vi "Spin pumping 83650B-2182-Kepco-475.vi"() -> ()   [LabVIEW 2020]
uses:
  <vilib>/Utility/file.llb/Write Delimited Spreadsheet (DBL).vi
panel:
  out "appended path":path
  in  "File Name":string
  in  "error out":errorcluster
  in  "stop":bool
  in  "Model 475 GPIB Addr":string="14"
  in  "Kepco GPIB Addr":string="6"
  in  "Model 2182 GPIB Addr":string="7"
  in  "83650B GPIB Addr":string="19"
  in  "Measurement Selection":T1(tab)
  out "History":cluster{dbl[], dbl[]}(graph)
  in  "Task":string[][](table)=[["1", "15", "8", "0.05", "2"]]
  out "Ongoing Measurement":cluster{dbl[], dbl[]}(graph)
  in  "Run":bool
  out "History 2":cluster{dbl[], dbl[]}(graph)
  in  "Task 2":string[][](table)=[["4", "1", "5", "0.05", "15", "10"]]
  out "Ongoing Measurement 2":cluster{dbl[], dbl[]}(graph)
  in  "Run 2":bool
  out "Field (Oe)":dbl
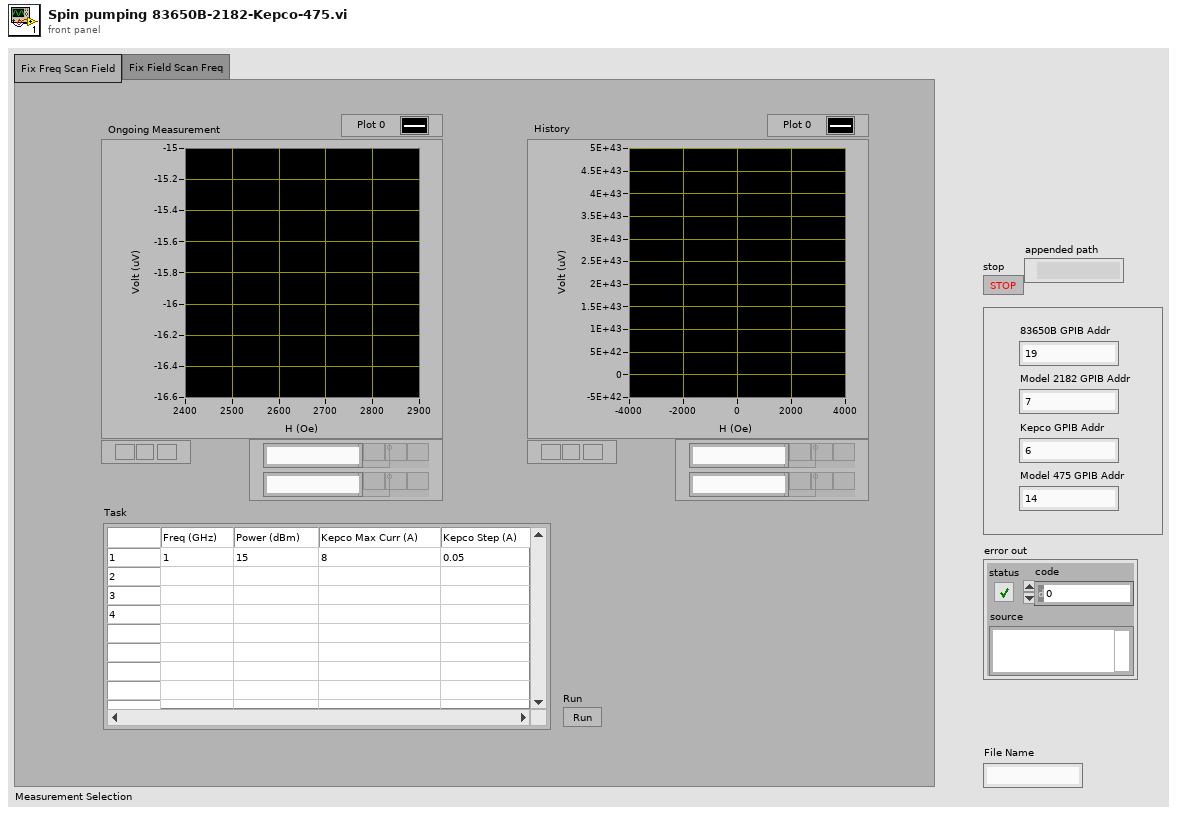
[diagram p1: front panel]
types:
  T1 = enum32{"Fix Freq Scan Field", "Fix Field Scan Freq"}
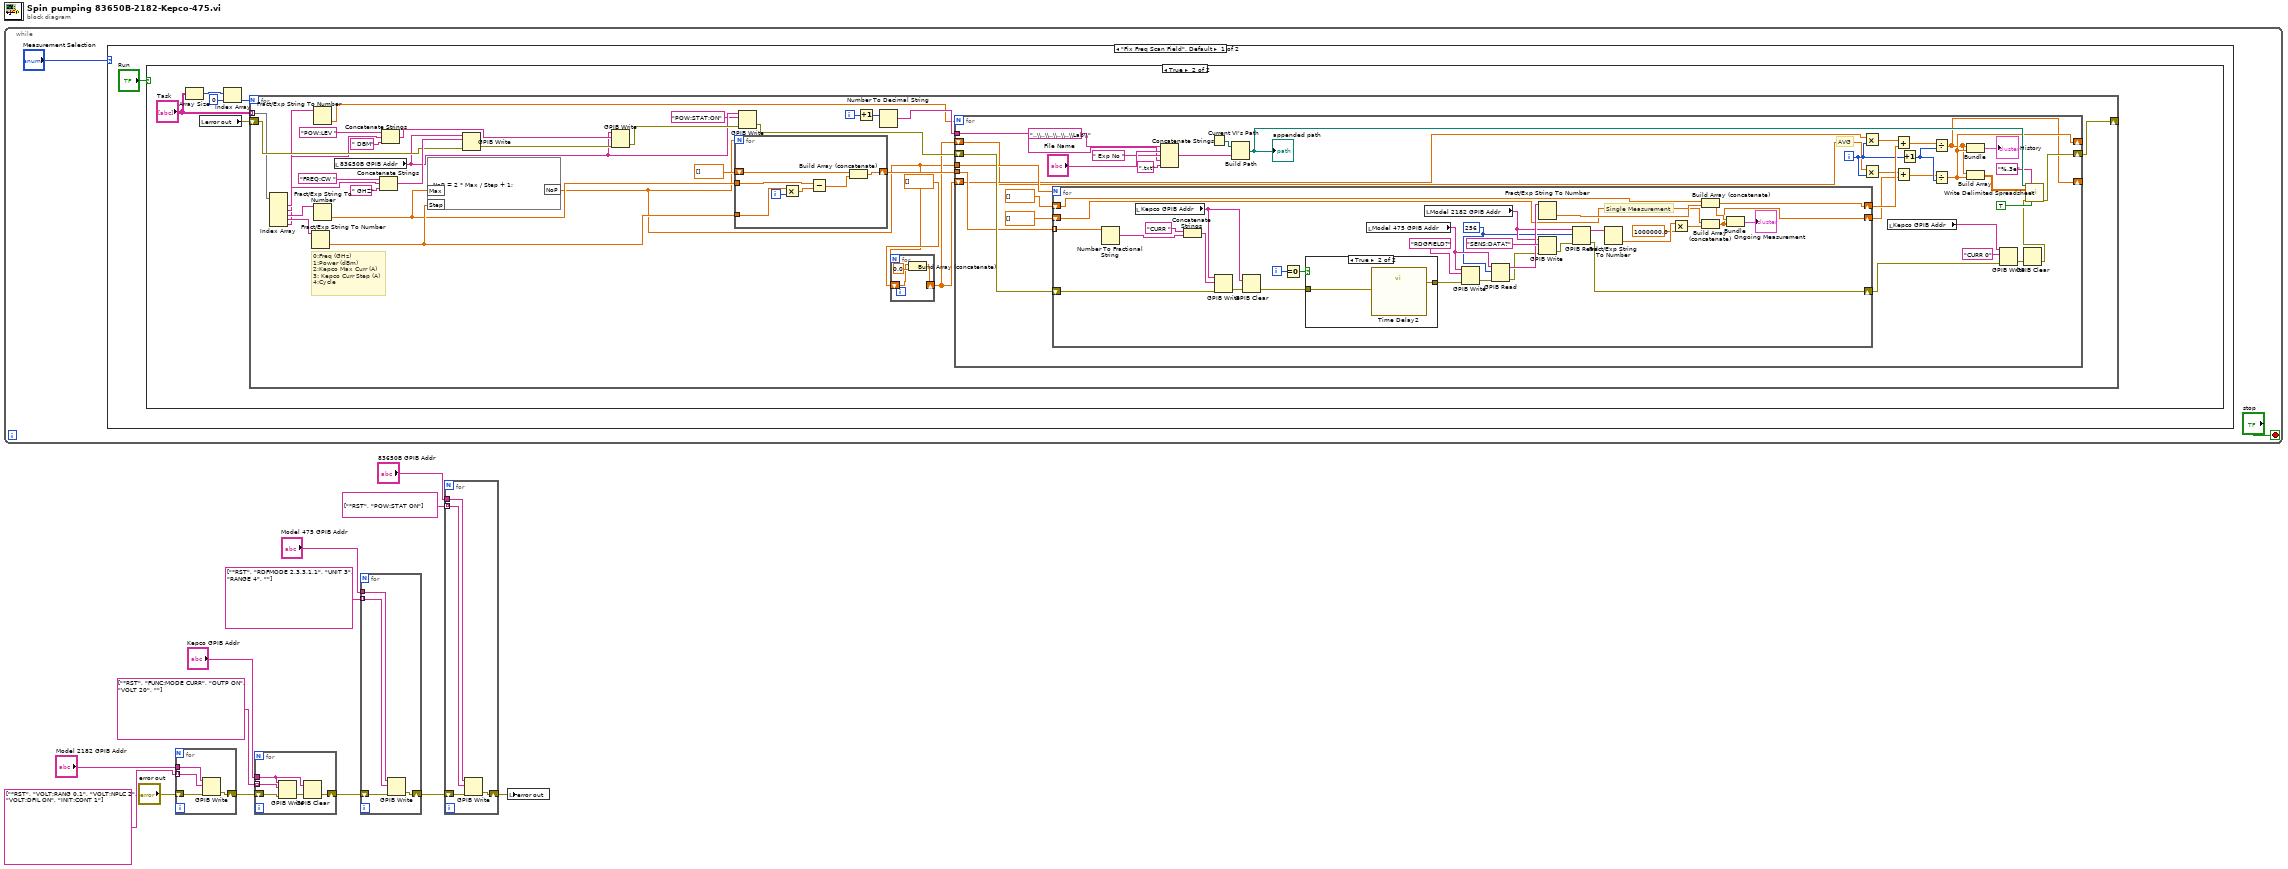
[diagram p0: block diagram]
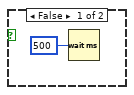
[diagram p2: hidden frame]
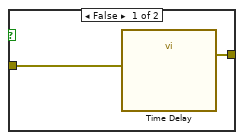
[diagram p3: hidden frame]
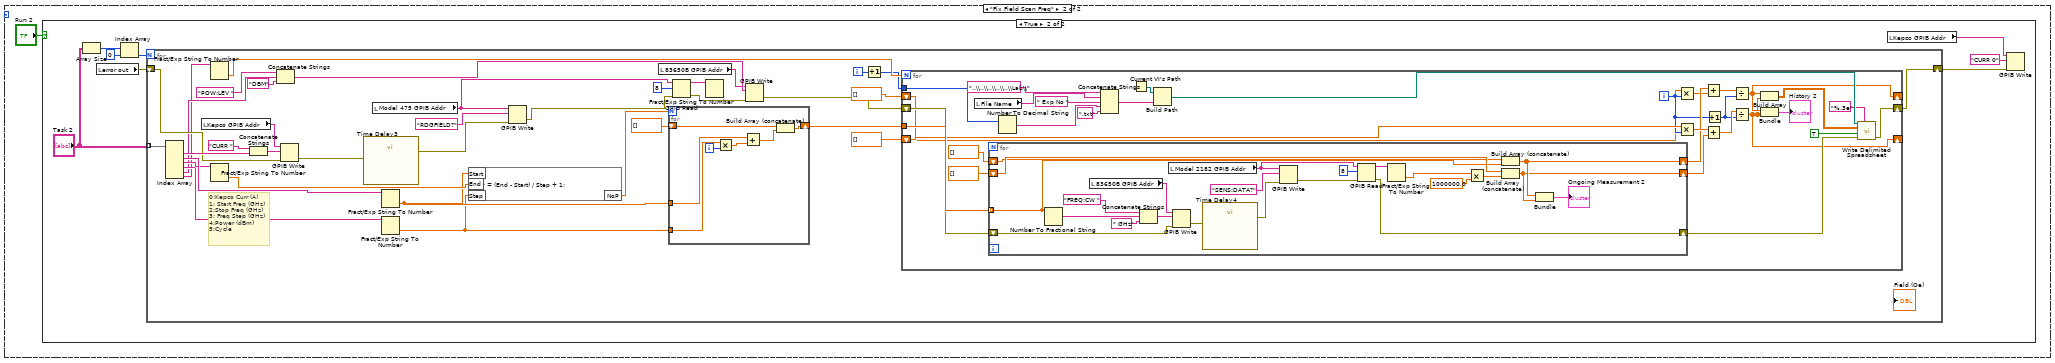
[diagram p4: hidden frame]
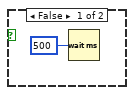
[diagram p5: hidden frame]
diagram:
  n1 = while {
    stop <- "stop" stop-if-true
    n2 = case shown="\"Fix Freq Scan Field\", Default" "Measurement Selection" {
      frame "Fix Freq Scan Field", Default {
        n3 = case shown="True" "Run" {
          frame False {
            n4 = Wait (ms)(milliseconds to wait=u32 500) -> ()  [unwired: 1 out]
          }
          frame True {
            n5 = Array Size(array="Task") -> (size(s)=w22:i32[])
            n6 = local read "error out"() -> (w18:errorcluster)
            n7 = Index Array(array=w22, index=0) -> (element=w21:i32)
            n8 = for {
              N: w21 -> [_]
              tunnel: "Task" -> [w40] mode=indexing
              shift-right: [w34] -> _
              shift-left: w18 -> [w42]
              i -> [w33]
              # "0:Freq (GHz)\n1:Power (dBm)\n2:Kepco Max Curr (A)\n3: Kepco Curr Step (A)\n4:Cycle"
              n9 = Index Array(array=w40) -> (element #1=w41:string, element #2=w39:string, element #3=w38:string, element #4=w37:string, element #5=w36:string)  [unwired: 5 in]
              n10 = Fract/Exp String To Number(string=w37) -> (number=w45:dbl)  [unwired: 3 in, 1 out]
              n11 = Fract/Exp String To Number(string=w36) -> (number=w26:dbl)  [unwired: 3 in, 1 out]
              n12 = Fract/Exp String To Number(string=w38) -> (number=w44:dbl)  [unwired: 3 in, 1 out]
              n13 = local read "83650B GPIB Addr"() -> (w28:string)
              n14 = Concatenate Strings("FREQ:CW " ("string"), w41, " GHZ" ("string")) -> (w48:string)
              n15 = Concatenate Strings("POW:LEV " ("string"), w39, " DBM" ("string")) -> (w50:string)
              n16 = formula code="NoP = 2 * Max / Step + 1;"("Max"=w44, "Step"=w45) -> ("NoP"=w23:dbl)
              n17 = GPIB Write(0:w28, 1:w48, 3:w42) -> (6:w49:errorcluster)  [unwired: 2 in, 1 out]
              n18 = GPIB Write(0:w28, 1:w50, 3:w49) -> (6:w29:errorcluster)  [unwired: 2 in, 1 out]
              n19 = for {
                N: w23 -> [_]
                shift-right: [w126] -> w35
                shift-left: dbl[] [] -> [w127]
                tunnel: w45 -> [w131]
                tunnel: w44 -> [w129]
                i -> [w132]
                n20 = Multiply(x=w131, y=w132) -> (x*y=w130:dbl)
                n21 = Subtract(x=w129, y=w130) -> (x-y=w128:dbl)
                n22 = Build Array (concatenate)(w127, w128) -> (w126:dbl[])
              }
              n23 = GPIB Write(0:w28, 1:"POW:STAT:ON" ("data"), 3:w29) -> (6:w30:errorcluster)  [unwired: 2 in, 1 out]
              n24 = Increment(x=w33) -> (x+1=w32:i32)
              n25 = Number To Decimal String(number=w32) -> (decimal integer string=w31:string)  [unwired: 1 in]
              n26 = for {
                N: w23 -> [_]
                shift-right: [w53] -> w24
                shift-left: dbl[] [] -> [w54]
                n27 = Build Array (concatenate)(w54, 0.0 ("element")) -> (w53:dbl[])
              }
              n28 = for {
                N: w26 -> [_]
                shift-right: [w81] -> w34
                shift-left: w30 -> [w84]
                tunnel: w35 -> [w83]
                tunnel: w23 -> [w82]
                shift-right: [w68] -> _
                shift-left: w24 -> [w77]
                shift-right: [w69] -> _
                shift-left: w24 -> [w72]
                tunnel: w31 -> [w63]
                i -> [w73]
                # "AVG"
                n29 = for {
                  N: w82 -> [_]
                  shift-right: [w102] -> w57
                  shift-left: w84 -> [w121]
                  tunnel: w83 -> [w119] mode=indexing
                  shift-right: [w101] -> w80
                  shift-left: dbl[] [] -> [w108]
                  shift-right: [w100] -> w75
                  shift-left: dbl[] [] -> [w104]
                  i -> [w114]
                  w106 = 256 ("byte count")
                  # "Single Measurement"
                  n30 = Number To Fractional String(number=w119) -> (F-format string=w118:string)  [unwired: 3 in]
                  n31 = local read "Kepco GPIB Addr"() -> (w91:string)
                  n32 = Concatenate Strings("CURR " ("string"), w118) -> (w117:string)
                  n33 = GPIB Write(0:w91, 1:w117, 3:w121) -> (6:w93:errorcluster)  [unwired: 2 in, 1 out]
                  n34 = GPIB Clear(2:w93, 3:w91) -> (0:w92:errorcluster)  [unwired: 1 out]
                  n35 = Equal To 0?(x=w114) -> (x = 0?=w113:bool)
                  n36 = case shown="True" w113 {
                    tunnel: w92 -> [w123 w125]
                    tunnel: [w122 w124] -> w115
                    frame False {
                      n37 = call "Time Delay"("error in (no error)"=w123) -> ("error out"=w122:errorcluster)  [unwired: 10 in]
                    }
                    frame True {
                      n38 = call "Time Delay2"("error in (no error)"=w125) -> ("error out"=w124:errorcluster)  [unwired: 10 in]
                    }
                  }
                  n39 = local read "Model 475 GPIB Addr"() -> (w111:string)
                  n40 = local read "Model 2182 GPIB Addr"() -> (w107:string)
                  n41 = GPIB Write(0:w111, 1:"RDGFIELD?" ("data"), 3:w115) -> (6:w95:errorcluster)  [unwired: 2 in, 1 out]
                  n42 = GPIB Read(0:w111, 1:w106, 3:w95) -> (5:w110:string, 7:w94:errorcluster)  [unwired: 2 in, 1 out]
                  n43 = Fract/Exp String To Number(string=w110) -> (number=w109:dbl)  [unwired: 3 in, 1 out]
                  n44 = GPIB Write(0:w107, 1:"SENS:DATA?" ("data"), 3:w94) -> (6:w103:errorcluster)  [unwired: 2 in, 1 out]
                  n45 = GPIB Read(0:w107, 1:w106, 3:w103) -> (5:w105:string, 7:w102:errorcluster)  [unwired: 2 in, 1 out]
                  n46 = Fract/Exp String To Number(string=w105) -> (number=w98:dbl)  [unwired: 3 in, 1 out]
                  n47 = Multiply(x=w98, y=1000000.0) -> (x*y=w96:dbl)
                  n48 = Build Array (concatenate)(w108, w109) -> (w101:dbl[])
                  n49 = Build Array (concatenate)(w104, w96) -> (w100:dbl[])
                  n50 = Bundle(w101, w100) -> (→"Ongoing Measurement":cluster{dbl[], dbl[]})  [unwired: 1 in]
                }
                n51 = Concatenate Strings("..\\..\\..\\..\\..\\Lab\\" ("string"), "File Name", " Exp No " ("string"), w63, ".txt" ("string")) -> (w88:string)
                n52 = Current VI's Path() -> (path=w62:path)
                n53 = Build Path(base path=w62, name or relative path=w88) -> (appended path=w89:path)
                "appended path" <- w89
                n54 = Multiply(x=w77, y=w73) -> (x*y=w79:dbl[])
                n55 = Multiply(x=w72, y=w73) -> (x*y=w74:dbl[])
                n56 = local read "Kepco GPIB Addr"() -> (w59:string)
                n57 = Add(x=w79, y=w80) -> (x+y=w78:dbl[])
                n58 = Add(x=w74, y=w75) -> (x+y=w71:dbl[])
                n59 = Increment(x=w73) -> (x+1=w76:i32)
                n60 = Divide(x=w78, y=w76) -> (x/y=w68:dbl[])
                n61 = Divide(x=w71, y=w76) -> (x/y=w69:dbl[])
                n62 = Bundle(w68, w69) -> (→"History":cluster{dbl[], dbl[]})  [unwired: 1 in]
                n63 = Build Array(w68, w69) -> (w67:dbl[][])
                n64 = GPIB Write(0:w59, 1:"CURR 0" ("data"), 3:w57) -> (6:w60:errorcluster)  [unwired: 2 in, 1 out]
                n65 = GPIB Clear(2:w60) -> (0:w56:errorcluster)  [unwired: 1 in, 1 out]
                n66 = call-poly <vilib>:"Write Delimited Spreadsheet.vi"("file path (dialog if empty)"=w89, "format (%.3f)"="%.3e", "2D data"=w67, "error in (no error)"=w56, "transpose? (no:F)"=TRUE) -> ("error out"=w81:errorcluster)  [unwired: 9 in, 1 out]
              }
            }
          }
        }
      }
      frame "Fix Field Scan Freq" {
        n67 = case shown="True" "Run 2" {
          frame False {
            n68 = Wait (ms)(milliseconds to wait=u32 500) -> ()  [unwired: 1 out]
          }
          frame True {
            n69 = Array Size(array="Task 2") -> (size(s)=w142:i32[])
            n70 = local read "error out"() -> (w138:errorcluster)
            n71 = Index Array(array=w142, index=0) -> (element=w140:i32)
            n72 = for {
              N: w140 -> [_]
              tunnel: "Task 2" -> [w178] mode=indexing
              shift-right: [w148] -> w137
              shift-left: w138 -> [w173]
              i -> [w147]
              # "0:Kepco Curr (A)\n1: Start Freq (GHz)\n2:Stop Freq (GHz)\n3: Freq Step (GHz)\n4:Power (dBm)\n5:Cycle"
              n73 = Index Array(array=w178) -> (element #1=w175:string, element #2=w171:string, element #3=w170:string, element #4=w169:string, element #5=w163:string, element #6=w158:string)  [unwired: 6 in]
              n74 = local read "Kepco GPIB Addr"() -> (w177:string)
              n75 = Fract/Exp String To Number(string=w158) -> (number=w157:dbl)  [unwired: 3 in, 1 out]
              n76 = Fract/Exp String To Number(string=w170) -> (number=w167:dbl)  [unwired: 3 in, 1 out]
              n77 = Concatenate Strings("CURR " ("string"), w175) -> (w174:string)
              n78 = Concatenate Strings("POW:LEV " ("string"), w163, "DBM" ("string")) -> (w160:string)
              n79 = GPIB Write(0:w177, 1:w174, 3:w173) -> (6:w172:errorcluster)  [unwired: 2 in, 1 out]
              n80 = call "Time Delay3"("error in (no error)"=w172) -> ("error out"=w154:errorcluster)  [unwired: 10 in]
              n81 = local read "Model 475 GPIB Addr"() -> (w152:string)
              n82 = Fract/Exp String To Number(string=w171) -> (number=w166:dbl)  [unwired: 3 in, 1 out]
              n83 = Fract/Exp String To Number(string=w169) -> (number=w165:dbl)  [unwired: 3 in, 1 out]
              n84 = formula code="NoP = (End - Start) / Step + 1;"("Start"=w166, "End"=w167, "Step"=w165) -> ("NoP"=w168:dbl)
              n85 = GPIB Write(0:w152, 1:"RDGFIELD?" ("data"), 3:w154) -> (6:w151:errorcluster)  [unwired: 2 in, 1 out]
              n86 = local read "83650B GPIB Addr"() -> (w145:string)
              n87 = for {
                N: w168 -> [_]
                shift-right: [w236] -> w159
                shift-left: dbl[] [] -> [w233]
                tunnel: w165 -> [w235]
                tunnel: w166 -> [w234]
                i -> [w239]
                n88 = Multiply(x=w235, y=w239) -> (x*y=w238:dbl)
                n89 = Add(x=w234, y=w238) -> (x+y=w237:dbl)
                n90 = Build Array (concatenate)(w233, w237) -> (w236:dbl[])
              }
              n91 = GPIB Read(0:w152, 1:8 ("byte count"), 3:w151) -> (5:w149:string, 7:w150:errorcluster)  [unwired: 2 in, 1 out]
              n92 = Fract/Exp String To Number(string=w149) -> ()  [unwired: 3 in, 2 out]
              n93 = GPIB Write(0:w145, 1:w160, 3:w150) -> (6:w143:errorcluster)  [unwired: 2 in, 1 out]
              n94 = Increment(x=w147) -> (x+1=w146:i32)
              n95 = for {
                N: w157 -> [_]
                tunnel: w159 -> [w209]
                shift-right: [w189] -> _
                shift-left: dbl[] [] -> [w204]
                shift-right: [w190] -> _
                shift-left: dbl[] [] -> [w197]
                shift-right: [w186] -> w148
                shift-left: w143 -> [w208]
                tunnel: w146 -> [w181]
                i -> [w198]
                n96 = local read "File Name"() -> (w192:string)
                n97 = for {
                  tunnel: w209 -> [w217] mode=indexing
                  shift-right: [w220] -> w191
                  shift-left: w208 -> [w228]
                  shift-right: [w213] -> w205
                  shift-left: dbl[] [] -> [w218]
                  shift-right: [w215] -> w200
                  shift-left: dbl[] [] -> [w216]
                  n98 = Number To Fractional String(number=w217) -> (F-format string=w231:string)  [unwired: 3 in]
                  n99 = local read "83650B GPIB Addr"() -> (w227:string)
                  n100 = Concatenate Strings("FREQ:CW " ("string"), w231, " GHz" ("string")) -> (w229:string)
                  n101 = local read "Model 2182 GPIB Addr"() -> (w223:string)
                  n102 = GPIB Write(0:w227, 1:w229, 3:w228) -> (6:w226:errorcluster)  [unwired: 2 in, 1 out]
                  n103 = call "Time Delay4"("error in (no error)"=w226) -> ("error out"=w224:errorcluster)  [unwired: 10 in]
                  n104 = GPIB Write(0:w223, 1:"SENS:DATA?" ("data"), 3:w224) -> (6:w221:errorcluster)  [unwired: 2 in, 1 out]
                  n105 = GPIB Read(0:w223, 1:8 ("byte count"), 3:w221) -> (5:w219:string, 7:w220:errorcluster)  [unwired: 2 in, 1 out]
                  n106 = Fract/Exp String To Number(string=w219) -> (number=w210:dbl)  [unwired: 3 in, 1 out]
                  n107 = Multiply(x=w210, y=1000000.0) -> (x*y=w212:dbl)
                  n108 = Build Array (concatenate)(w216, w217) -> (w215:dbl[])
                  n109 = Build Array (concatenate)(w218, w212) -> (w213:dbl[])
                  n110 = Bundle(w215, w213) -> (→"Ongoing Measurement 2":cluster{dbl[], dbl[]})  [unwired: 1 in]
                }
                n111 = Number To Decimal String(number=w181) -> (decimal integer string=w183:string)  [unwired: 1 in]
                n112 = Concatenate Strings("..\\..\\..\\..\\..\\Lab\\" ("string"), w192, " Exp No " ("string"), w183, ".txt" ("string")) -> (w194:string)
                n113 = Current VI's Path() -> (path=w180:path)
                n114 = Build Path(base path=w180, name or relative path=w194) -> (appended path=w193:path)
                n115 = Multiply(x=w197, y=w198) -> (x*y=w199:dbl[])
                n116 = Multiply(x=w204, y=w198) -> (x*y=w203:dbl[])
                n117 = Add(x=w200, y=w199) -> (x+y=w201:dbl[])
                n118 = Add(x=w203, y=w205) -> (x+y=w202:dbl[])
                n119 = Increment(x=w198) -> (x+1=w184:i32)
                n120 = Divide(x=w201, y=w184) -> (x/y=w190:dbl[])
                n121 = Divide(x=w202, y=w184) -> (x/y=w189:dbl[])
                n122 = Build Array(w190, w189) -> (w188:dbl[][])
                n123 = Bundle(w190, w189) -> (→"History 2":cluster{dbl[], dbl[]})  [unwired: 1 in]
                n124 = call-poly <vilib>:"Write Delimited Spreadsheet.vi"("file path (dialog if empty)"=w193, "format (%.3f)"="%.3e", "2D data"=w188, "append to file? (new file:F)"=TRUE ("transpose? (no:F)"), "error in (no error)"=w191) -> ("error out"=w186:errorcluster)  [unwired: 9 in, 1 out]
              }
            }
            n125 = local read "Kepco GPIB Addr"() -> (w136:string)
            n126 = GPIB Write(0:w136, 1:"CURR 0" ("data"), 3:w137) -> ()  [unwired: 2 in, 2 out]
          }
        }
      }
    }
  }
  n127 = for {
    tunnel: "Model 2182 GPIB Addr" -> [w243]
    tunnel: string[] ["*RST", "VOLT:RANG 0.1", "VOLT:NPLC 2", "VOLT:DFIL ON", "INIT:CONT 1"] -> [w242] mode=indexing
    shift-right: [w241] -> w7
    shift-left: "error out" -> [w240]
    n128 = GPIB Write(0:w243, 1:w242, 3:w240) -> (6:w241:errorcluster)  [unwired: 2 in, 1 out]
  }
  n129 = for {
    tunnel: "Kepco GPIB Addr" -> [w244]
    tunnel: string[] ["*RST", "FUNC:MODE CURR", "OUTP ON", "VOLT 20", ""] -> [w248] mode=indexing
    shift-right: [w245] -> w6
    shift-left: w7 -> [w247]
    n130 = GPIB Write(0:w244, 1:w248, 3:w247) -> (6:w246:errorcluster)  [unwired: 2 in, 1 out]
    n131 = GPIB Clear(2:w246, 3:w244) -> (0:w245:errorcluster)  [unwired: 1 out]
  }
  n132 = for {
    tunnel: "Model 475 GPIB Addr" -> [w252]
    tunnel: string[] ["*RST", "RDFMODE 2,3,3,1,1", "UNIT 3", "RANGE 4", ""] -> [w251] mode=indexing
    shift-right: [w250] -> w3
    shift-left: w6 -> [w249]
    n133 = GPIB Write(0:w252, 1:w251, 3:w249) -> (6:w250:errorcluster)  [unwired: 2 in, 1 out]
  }
  n134 = for {
    tunnel: "83650B GPIB Addr" -> [w256]
    tunnel: string[] ["*RST", "POW:STAT ON"] -> [w255] mode=indexing
    shift-right: [w253] -> w2
    shift-left: w3 -> [w254]
    n135 = GPIB Write(0:w256, 1:w255, 3:w254) -> (6:w253:errorcluster)  [unwired: 2 in, 1 out]
  }
  n136 = local write "error out"(w2) -> ()
